vi "Global.vi"() -> ()   [LabVIEW 2015]
panel:
  out "Run":bool
  out "Rec":variant
  out "EOS":bool
  in  "VARS":T1(array[cluster])=[{"VAR"="HOLD", "Options"="", "Val"="", "Recieved"=TRUE, "Set"=FALSE}]
  in  "Trigger":dbl format="%#_13g"
  out "Acquire":bool
  out "H5":path[](array[path])
  out "Save":bool
  out "SEQLine":string="END"
  out "RID":string
  out "SQUID":string="3"
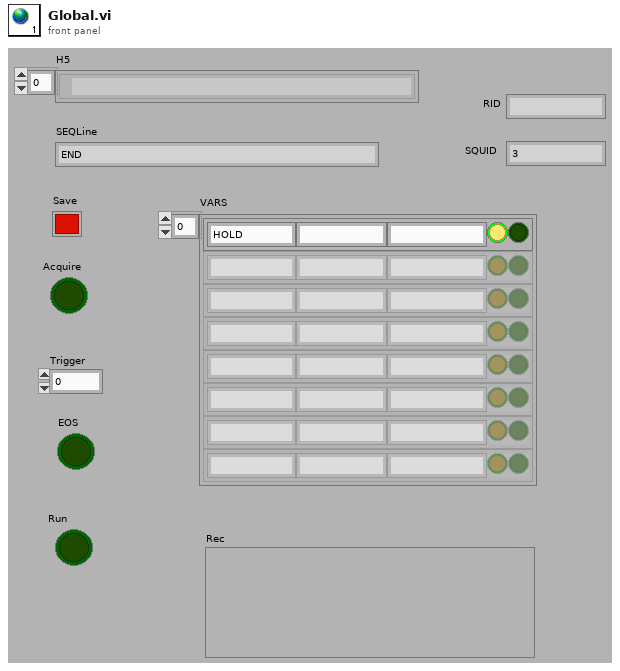
[diagram p1: front panel]
types:
  T1 = cluster{"VAR":string, "Options":string, "Val":string, "Recieved":bool, "Set":bool}[]
diagram:
